vi "Transpose.vi"   [LabVIEW 2014]
uses:
  <vilib>/Utility/file.llb/Read From Spreadsheet File (DBL).vi
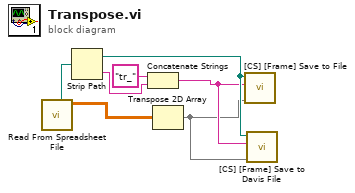
[diagram p0: block diagram]
diagram:
  n1 = call-poly <vilib>:"Read From Spreadsheet File.vi"() -> ("all rows"=w7:dbl[][], "new file path (Not A Path if cancelled)"=w6:path)  [unwired: 7 in, 3 out]
  n2 = Strip Path(path=w6) -> (stripped path=w3:path, name=w4:string)
  n3 = Concatenate Strings("tr_" ("string"), w4) -> (w2:string)
  n4 = Transpose 2D Array(2D array=w7) -> (transposed array=w1:dbl[][])
  n5 = call "[CS] [Frame] Save to File.vi"("array"=w1, "Name"=w2, "base path"=w3) -> ()  [unwired: 9 in]
  n6 = call "[CS] [Frame] Save to Davis File.vi"("array"=w1, "Name"=w2, "base path"=w3) -> ()  [unwired: 9 in]
